vi "Helmholtz2D_Check Input_Domain.vi"(8 "error in (no error)":errorcluster, 11 "Domain":T1={"x"={"start x"=0.0, "end x"=1.0, "# of x-points"=11}, "y"={"start y"=0.0, "end y"=1.0, "# of y-points"=11}}) -> (0 "error out":errorcluster)   [LabVIEW 2017, in "NI_PDE.lvlib"]
uses:
  <vilib>/gmath/NI_PDE.lvlib
  <vilib>/gmath/pde.llb/Common/PDE_Error.ctl
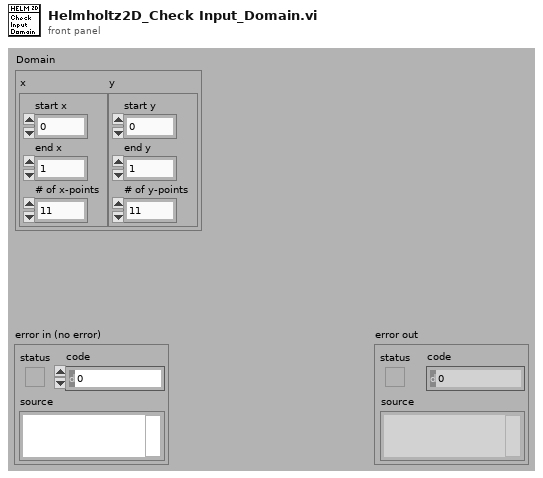
[diagram p1: front panel]
types:
  T1 = cluster{"x":cluster{"start x":dbl, "end x":dbl, "# of x-points":i32}, "y":cluster{"start y":dbl, "end y":dbl, "# of y-points":i32}}
  T2 = typedef "NI_PDE.lvlib/PDE_Error.ctl" = enum16{"No Error", "k is zero", "End point <= start point", "# of time steps < 2", "# of spatial points < 3", "# of grid < 1 for FEM", "# of boundary < 3 for FEM", "Incompatible RHS size", "Incompatible BC size", "Incompatible IC size", "PDE class conflict", "RHS class conflict", "Domain class conflict", "BC class conflict", "IC class conflict"}
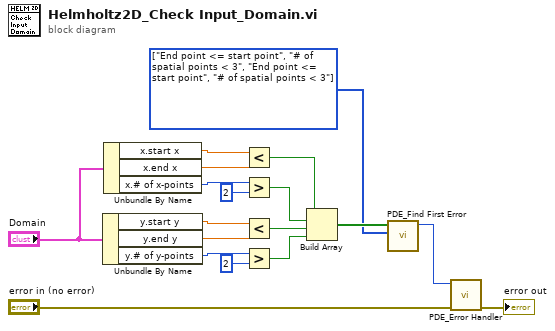
[diagram p0: block diagram]
diagram:
  w1 = T2[] [enum."End point <= start point", enum."# of spatial points < 3", enum."End point <= start point", enum."# of spatial points < 3"] items=["No Error", "k is zero", "End point <= start point", "# of time steps < 2", "# of spatial points < 3", "# of grid < 1 for FEM", "# of boundary < 3 for FEM", "Incompatible RHS size", "Incompatible BC size", "Incompatible IC size", "PDE class conflict", "RHS class conflict", "Domain class conflict", "BC class conflict", "IC class conflict"]
  n1 = Unbundle By Name("Domain") -> ("y.start y"=w11:dbl, "y.end y"=w12:dbl, "y.# of y-points"=w13:i32)
  n2 = Unbundle By Name("Domain") -> ("x.start x"=w18:dbl, "x.end x"=w17:dbl, "x.# of x-points"=w16:i32)
  n3 = Less?(x=w18, y=w17) -> (x < y?=w9:bool)
  n4 = Greater?(x=w16, y=2) -> (0:w8:bool)
  n5 = Less?(x=w11, y=w12) -> (x < y?=w7:bool)
  n6 = Greater?(x=w13, y=2) -> (0:w6:bool)
  n7 = Build Array(w9, w8, w7, w6) -> (w3:bool[])
  n8 = call <vilib>:"PDE_Find First Error.vi"("PDE Error"=w1, "Failure"=w3) -> ("first error"=w2:T2)  [unwired: 9 out]
  n9 = call <vilib>:"PDE_Error Handler.vi"("error in (no error)"="error in (no error)", "PDE error"=w2) -> ("error out"=→"error out":errorcluster)  [unwired: 9 out]
